vi "Cannon Angle Set.vi"(8 "set angle 0 to be min angle":bool, 11 "Angle Set Point":dbl(knob) scale=0.0..200.0) -> (2 "On Target":bool, 3 "zAvit Vbus Out":dbl)   [LabVIEW 2012]
uses:
  BotStatus.vi
panel:
  # "Cannon Angle"
  # "90-min / 90"
  # "0 / min angle"
  # "90 / min+90"
  # "T / F"
  # "-min angle / 0"
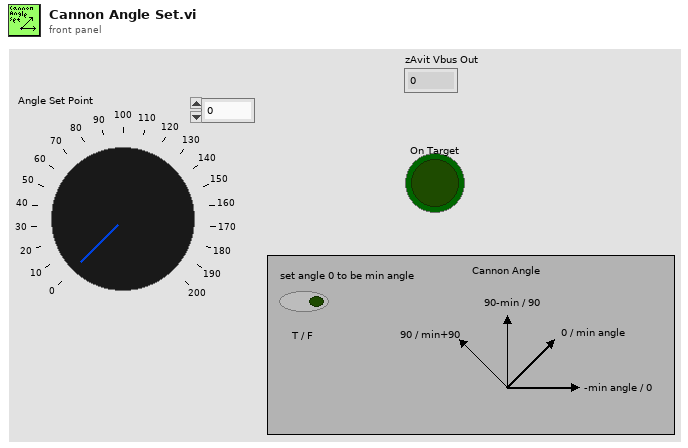
[diagram p1: front panel]
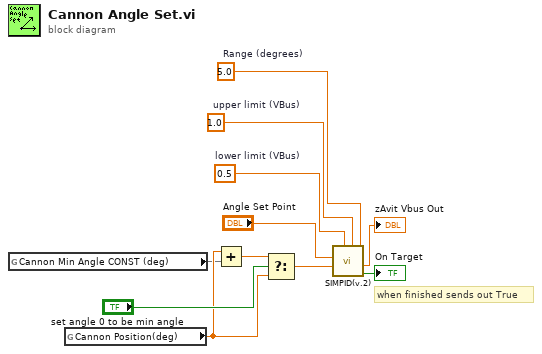
[diagram p0: block diagram]
diagram:
  w11 = 0.5  # lower limit (VBus)
  w10 = 1.0  # upper limit (VBus)
  w9 = 5.0  # Range (degrees)
  # "when finished sends out True"
  n1 = global read "BotStatus.vi" "Cannon Min Angle CONST (deg)"() -> (w2)
  n2 = global read "BotStatus.vi" "Cannon Position(deg)"() -> (w3:dbl)
  n3 = Add(x=w3, y=w2) -> (x+y=w1:dbl)
  n4 = Select(t=w1, s="set angle 0 to be min angle", f=w3) -> (s? t:f=w4:dbl)
  n5 = call "SIMPID(v.2).vi"("Range"=w9, "upper limit"=w10, "lower limit"=w11, "Current Point"=w4, "Set Point"="Angle Set Point") -> ("On Target"=→"On Target":bool, "result"=→"zAvit Vbus Out":dbl)  [unwired: 5 in]
